vi "Build Tag Name.vi"(10 "Resource":string, 11 "Tag":string) -> (3 "System Tag":string)   [LabVIEW 2016]
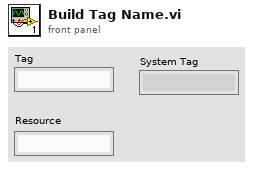
[diagram p1: front panel]
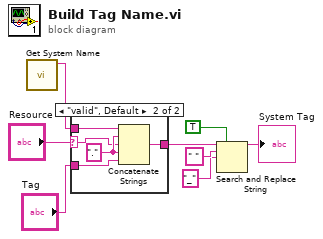
[diagram p0: block diagram]
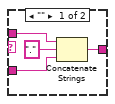
[diagram p2: hidden frame]
diagram:
  n1 = call "Get System Name.vi"() -> ("System Name"=w1:string)  [unwired: 11 in]
  n2 = case shown="\"valid\", Default" "Resource" {
    selector: "Resource" -> [_ w13]
    tunnel: [w9 w17] -> w5
    tunnel: w1 -> [w12 w16]
    tunnel: "Tag" -> [w11 w15]
    frame "" {
      n3 = Concatenate Strings(w12, "." ("element"), w11) -> (w9:string)
    }
    frame "valid", Default {
      w14 = "." ("element")
      n4 = Concatenate Strings(w16, w14, w13, w14, w15) -> (w17:string)
    }
  }
  n5 = Search and Replace String(replace all?=TRUE ("replace all? (F)"), input string=w5, search string=" ", replace string="_" ("replace string (\"\")")) -> (result string=→"System Tag":string)  [unwired: 4 in, 3 out]
